vi "GetWelcome.vi"(3 "error in (no error)":errorcluster, 5 "TCP Network Connection in":refnum<k5>) -> (0 "error out":errorcluster, 1 "TCP Network Connection out":refnum<k5>, 2 "data out":string)   [LabVIEW 2013]
panel:
  out "Msg Type":i32
  out "Msg Size":i32
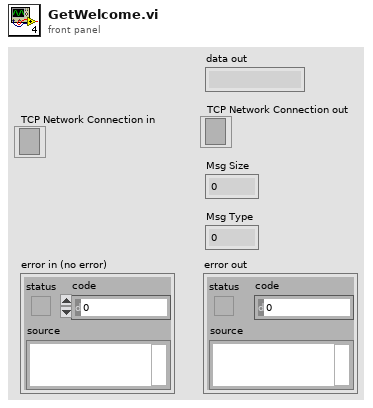
[diagram p1: front panel]
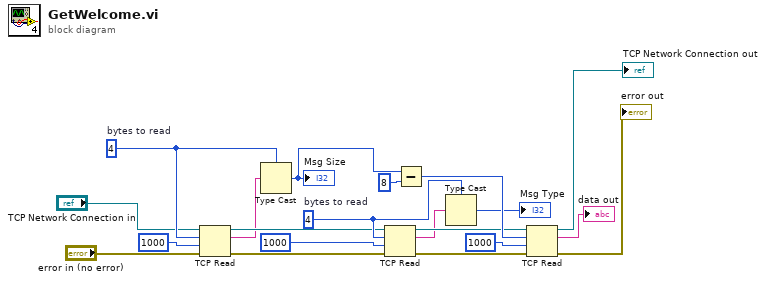
[diagram p0: block diagram]
diagram:
  w9 = 4  # bytes to read
  w6 = 4  # bytes to read
  n1 = TCP Read(connection ID="TCP Network Connection in", bytes to read=w6, error in (no error)="error in (no error)", 9:1000 ("timeout ms (25000)")) -> (connection ID out=w4:refnum<k5>, data out=w3:string, error out=w5:errorcluster)  [unwired: 1 in]
  n2 = Type Cast(type=w6, x=w3) -> (*(type *) &x=w14:i32)
  "Msg Size" <- w14
  n3 = TCP Read(connection ID=w4, bytes to read=w9, error in (no error)=w5, 9:1000 ("timeout ms (25000)")) -> (connection ID out=w12:refnum<k5>, data out=w11:string, error out=w13:errorcluster)  [unwired: 1 in]
  n4 = Subtract(x=w14, y=8) -> (x-y=w16:i32)
  n5 = Type Cast(type=w9, x=w11) -> (*(type *) &x=→"Msg Type":i32)
  n6 = TCP Read(connection ID=w12, bytes to read=w16, error in (no error)=w13, 9:1000 ("timeout ms (25000)")) -> (connection ID out=→"TCP Network Connection out":refnum<k5>, data out=→"data out":string, error out=→"error out":errorcluster)  [unwired: 1 in]
